vi "output.vi"(8 "error in":errorcluster, 10 "data table in":T1, 11 "FPGA Module runtime in":refnum<class "FPGA Module runtime.lvclass">) -> (0 "error out":errorcluster, 2 "data table out":T1, 3 "FPGA Module runtime out":refnum<class "FPGA Module runtime.lvclass">)   [LabVIEW 2017, in "FPGA Module runtime.lvclass"]
doc: "Provides an interface for writing data to a module at runtime. While this interface performs no operations, a child should provide an override which may write to any open sessions, references, or interfaces."
uses:
  FPGA Module runtime.lvclass
  <vilib>/NI/Tag Bus/table/data table.ctl
  FPGA Module runtime.lvclass/FPGA Module runtime.ctl
  OLD Project Folder/fpga channel/FXP I_20_5.ctl
  OLD Project Folder/fpga channel/FXP I_24_5.ctl
  OLD Project Folder/fpga channel/FXP I_24_10.ctl
  <vilib>/NI/Tag Bus/table/data polymorphs/read many/read Doubles.vi
  <vilib>/NI/Tag Bus/table/data polymorphs/read many/read Singles.vi
  <vilib>/NI/Tag Bus/table/data polymorphs/read many/read I64s.vi
  <vilib>/NI/Tag Bus/table/data polymorphs/read many/read I32s.vi
  <vilib>/NI/Tag Bus/table/data polymorphs/read many/read I16s.vi
  <vilib>/NI/Tag Bus/table/data polymorphs/read many/read I8s.vi
  <vilib>/NI/Tag Bus/table/data polymorphs/read many/read U64s.vi
  <vilib>/NI/Tag Bus/table/data polymorphs/read many/read U32s.vi
  <vilib>/NI/Tag Bus/table/data polymorphs/read many/read U16s.vi
  <vilib>/NI/Tag Bus/table/data polymorphs/read many/read U8s.vi
  <vilib>/NI/Tag Bus/table/data polymorphs/read many/read Booleans.vi
  <vilib>/NI/Tag Bus/table/data polymorphs/read many/read Array of Booleans.vi
  <vilib>/NI/Tag Bus/table/data polymorphs/read one/read Array of Double.vi
  <vilib>/NI/Tag Bus/table/data polymorphs/read one/read Array of Single.vi
  <vilib>/NI/Tag Bus/table/data polymorphs/read one/read Array of I64.vi
  <vilib>/NI/Tag Bus/table/data polymorphs/read one/read Array of I32.vi
  <vilib>/NI/Tag Bus/table/data polymorphs/read one/read Array of I16.vi
  <vilib>/NI/Tag Bus/table/data polymorphs/read one/read Array of I8.vi
  <vilib>/NI/Tag Bus/table/data polymorphs/read one/read Array of U64.vi
  <vilib>/NI/Tag Bus/table/data polymorphs/read one/read Array of U32.vi
  <vilib>/NI/Tag Bus/table/data polymorphs/read one/read Array of U16.vi
  <vilib>/NI/Tag Bus/table/data polymorphs/read one/read Array of U8.vi
  <vilib>/Utility/error.llb/Error Cluster From Error Code.vi
  <vilib>/rvi/errors/niLvFpgaAdjustHostInterfaceError.vi
  <vilib>/rvi/interface/nirviReadWriteControl/nirviReadWriteControl.xnode
  <vilib>/NI/Tag Bus/table/data table.lvlib
  fpga channel/FPGA Channel.lvclass
  NiFpgaLv.dll
  <vilib>/rvi/interface/Simulation/niFpgaSimulationCallBeginRW.vi
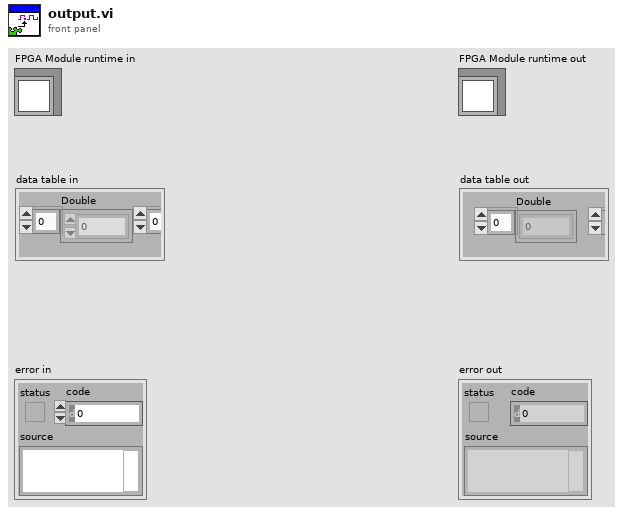
[diagram p1: front panel]
types:
  T1 = typedef "tag bus.lvlib/data table.lvlib/data table.ctl" = cluster{"Double":dbl[], "Single":sgl[], "I64":i64[], "I32":i32[], "I16":i16[], "I8":i8[], "U64":u64[], "U32":u32[], "U16":u16[], "U8":u8[], "Boolean":bool[], "String":string[], "Array of Double":cluster{"DBL Array":dbl[]}[], "Array of Single":cluster{"SGL Array":sgl[]}[], "Array of I64":cluster{"I64 Array":i64[]}[], "Array of I32":cluster{"I32 Array":i32[]}[], "Array of I16":cluster{"I16 Array":i16[]}[], "Array of I8":cluster{"I8 Array":i8[]}[], "Array of U64":cluster{"U64 Array":u64[]}[], "Array of U32":cluster{"U32 Array":u32[]}[], "Array of U16":cluster{"U16 Array":u16[]}[], "Array of U8":cluster{"U8 Array":u8[]}[], "Array of Boolean":cluster{"Boolean Array":bool[]}[], "Array of String":cluster{"String Array":string[]}[]}
  T2 = typedef "FPGA Module runtime.lvclass/ControlsMappings.ctl" = cluster{"data type":T3, "fpga res type":T4[], "fpga resource":refnum<k20>[], "data indexes":i32[]}
  T3 = typedef "tag bus.lvlib/tag descriptor.lvclass/Data Type.ctl" = enum16{"Double", "Single", "I64", "I32", "I16", "I8", "U64", "U32", "U16", "U8", "Boolean", "String", "Array of Double", "Array of Single", "Array of I64", "Array of I32", "Array of I16", "Array of I8", "Array of U64", "Array of U32", "Array of U16", "Array of U8", "Array of Boolean", "Array of String"}
  T4 = typedef "FPGA Channel.lvclass/fpga resource supported data types.ctl" = enum16{"Invalid Type", "Single", "I64", "I32", "I16", "I8", "U64", "U32", "U16", "U8", "Boolean", "FXP I,20,5", "FXP I,24,5", "FXP I,24,10", "Fifo 1023,I16"}
  T5 = typedef "FPGA Channel.lvclass/FXP I_20_5.ctl" = refnum<k20>
  T6 = typedef "FPGA Channel.lvclass/FXP I_24_5.ctl" = refnum<k20>
  T7 = typedef "FPGA Channel.lvclass/FXP I_24_10.ctl" = refnum<k20>
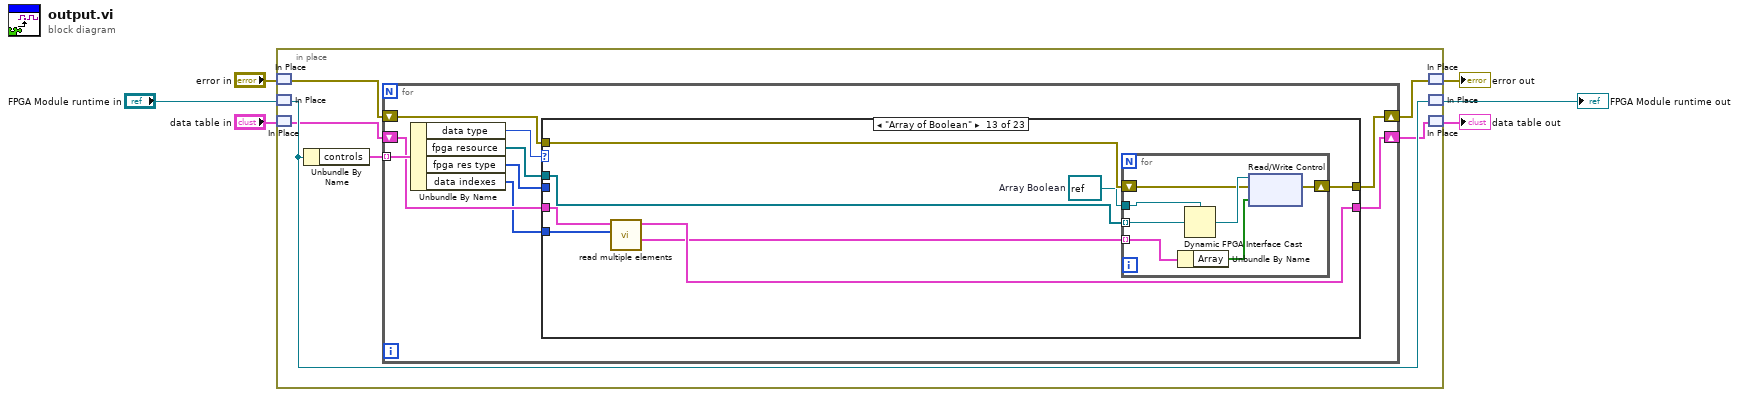
[diagram p0: block diagram]
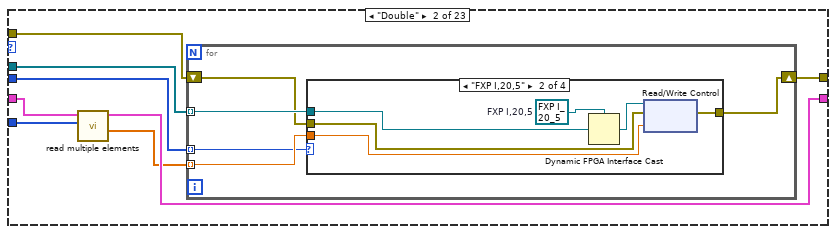
[diagram p3: hidden frame]
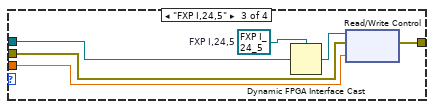
[diagram p5: hidden frame]
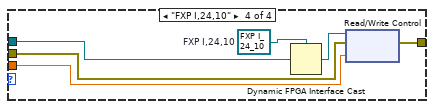
[diagram p6: hidden frame]
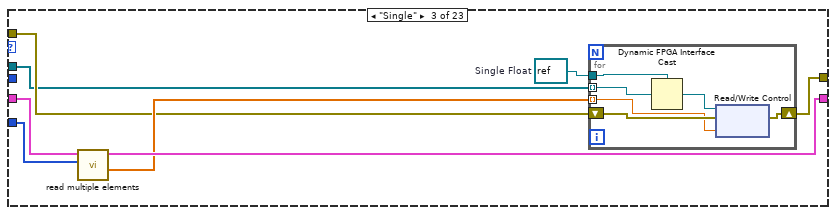
[diagram p7: hidden frame]
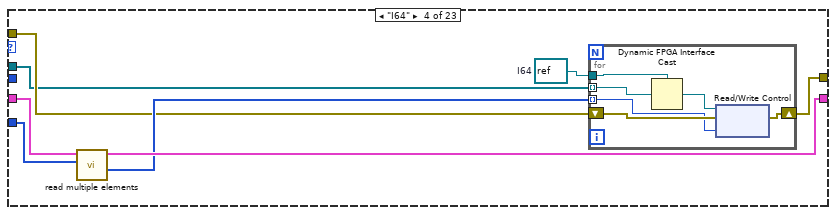
[diagram p8: hidden frame]
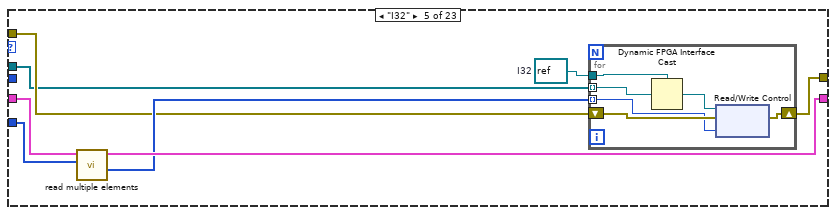
[diagram p9: hidden frame]
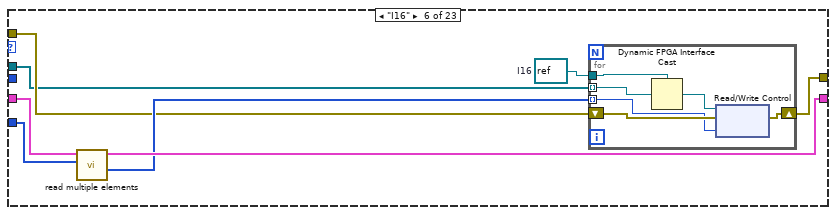
[diagram p10: hidden frame]
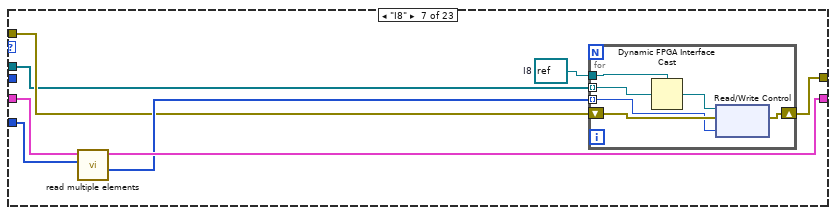
[diagram p11: hidden frame]
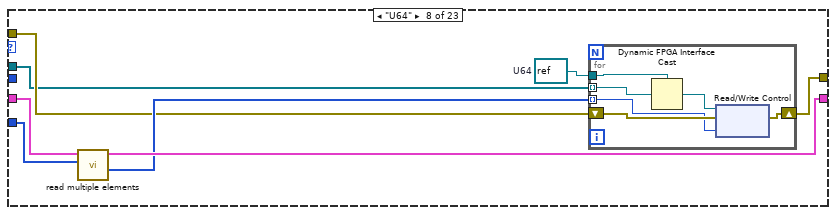
[diagram p12: hidden frame]
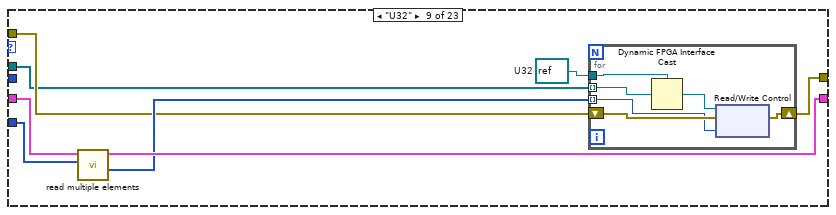
[diagram p13: hidden frame]
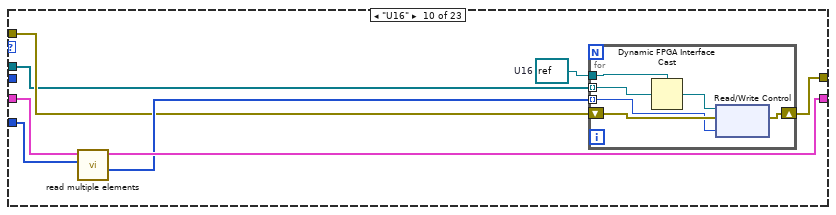
[diagram p14: hidden frame]
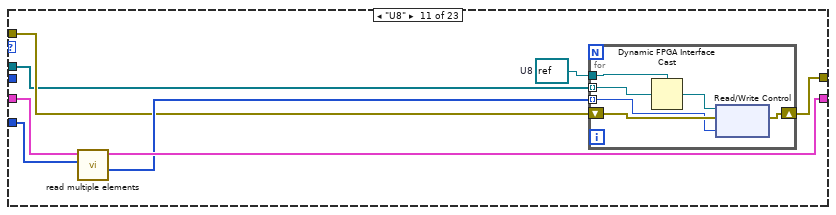
[diagram p15: hidden frame]
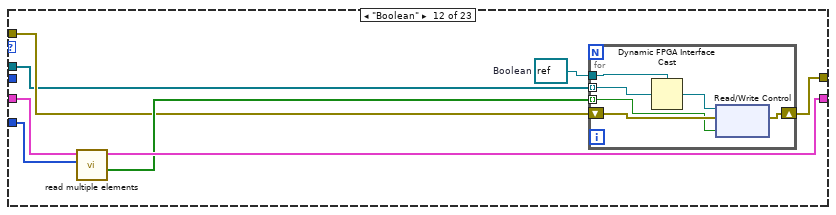
[diagram p16: hidden frame]
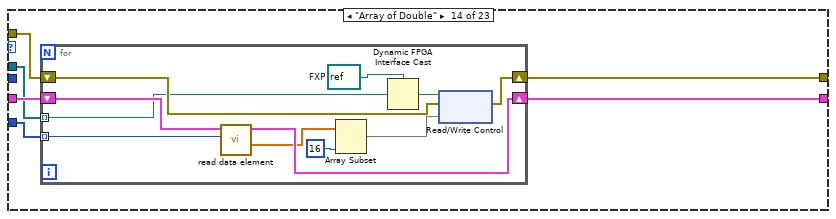
[diagram p17: hidden frame]
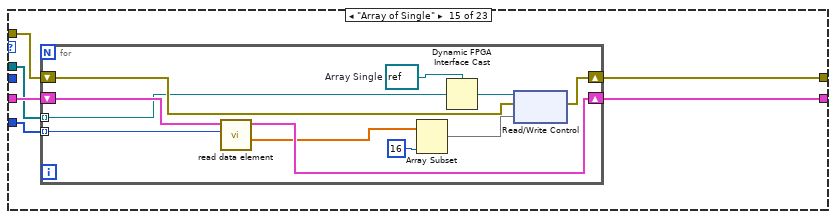
[diagram p18: hidden frame]
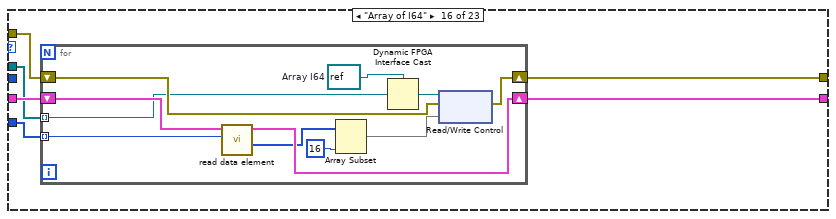
[diagram p19: hidden frame]
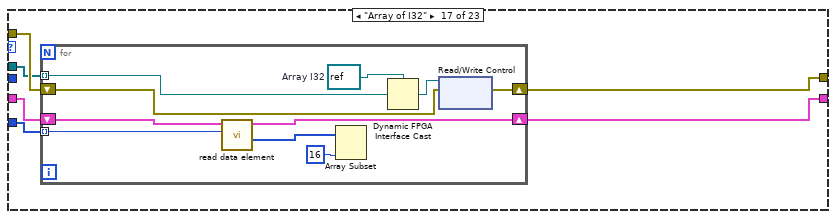
[diagram p20: hidden frame]
diagram:
  n1 = in-place {
    n2 = in-place-match #1("error in") -> (w7:errorcluster)
    n3 = in-place-match #2("FPGA Module runtime in") -> (w11:refnum<class "FPGA Module runtime.lvclass">)
    n4 = in-place-match #3("data table in") -> (w10:T1)
    n5 = Unbundle By Name(w11) -> ("controls"=w12:T2[])
    n6 = for {
      shift-right: [w20] -> w9
      shift-left: w10 -> [w19]
      shift-right: [w15] -> w8
      shift-left: w7 -> [w18]
      tunnel: w12 -> [w21] mode=indexing
      n7 = Unbundle By Name(w21) -> ("data type"=w14:T3, "fpga resource"=w16:refnum<k20>[], "fpga res type"=w13:T4[], "data indexes"=w17:i32[])
      n8 = case shown="\"Array of Boolean\"" w14 {
        tunnel: [w23 w30 w62 w76 w90 w104 w118 w132 w146 w160 w174 w188 w202 w215 w232 w249 w266 w282 w299 w316 w333 w350 w367] -> w20
        tunnel: w19 -> [w23 w31 w63 w77 w91 w105 w119 w133 w147 w161 w175 w189 w203 w216 w233 w250 w267 w283 w300 w317 w334 w351 w368]
        tunnel: w18 -> [w22 w27 w59 w73 w87 w101 w115 w129 w143 w157 w171 w185 w199 w213 w230 w247 w264 w280 w297 w314 w331 w348 w365]
        tunnel: w17 -> [_ w29 w61 w75 w89 w103 w117 w131 w145 w159 w173 w187 w201 w214 w231 w248 w265 w281 w298 w315 w332 w349 w366]
        tunnel: w16 -> [_ w26 w58 w72 w86 w100 w114 w128 w142 w156 w170 w184 w198 w212 w229 w246 w263 w279 w296 w313 w330 w347 w364]
        tunnel: [w22 w25 w56 w70 w84 w98 w112 w126 w140 w154 w168 w182 w197 w211 w228 w245 w262 w278 w295 w312 w329 w346 w363] -> w15
        tunnel: w13 -> [_ w24 _ _ _ _ _ _ _ _ _ _ _ _ _ _ _ _ _ _ _ _ _]
        frame Default {
        }
        frame "Double" {
          n9 = call-poly <vilib>:"read multiple elements.vi"("indices"=w29, "data table in"=w31) -> ("values"=w28:dbl[], "data table out"=w30:T1)  [unwired: 8 in]
          n10 = for {
            tunnel: w26 -> [w36] mode=indexing
            shift-right: [w34] -> w25
            shift-left: w27 -> [w35]
            tunnel: w28 -> [w33] mode=indexing
            tunnel: w24 -> [w32] mode=indexing
            n11 = case shown="\"FXP I,20,5\"" w32 {
              tunnel: w36 -> [_ w43 w49 w55]
              tunnel: w35 -> [w37 w41 w47 w53]
              tunnel: [w37 w40 w46 w52] -> w34
              tunnel: w33 -> [_ w39 w45 w51]
              frame "Invalid Type", Default {
              }
              frame "FXP I,20,5" {
                w38 = T5 refnum  # FXP I,20,5
                n12 = Dynamic FPGA Interface Cast(Session In=w38, Type=w43) -> (Session Out=w42:T5)
                n13 = xnode "Read/Write Control"("FPGA VI Reference In"=w42, "error in"=w41, "Value"=w39) -> ("error out"=w40:errorcluster)  [unwired: 1 out]
              }
              frame "FXP I,24,5" {
                w44 = T6 refnum  # FXP I,24,5
                n14 = Dynamic FPGA Interface Cast(Session In=w44, Type=w49) -> (Session Out=w48:T6)
                n15 = xnode "Read/Write Control"("FPGA VI Reference In"=w48, "error in"=w47, "Value"=w45) -> ("error out"=w46:errorcluster)  [unwired: 1 out]
              }
              frame "FXP I,24,10" {
                w50 = T7 refnum  # FXP I,24,10
                n16 = Dynamic FPGA Interface Cast(Session In=w50, Type=w55) -> (Session Out=w54:T7)
                n17 = xnode "Read/Write Control"("FPGA VI Reference In"=w54, "error in"=w53, "Value"=w51) -> ("error out"=w52:errorcluster)  [unwired: 1 out]
              }
            }
          }
        }
        frame "Single" {
          w57 = refnum<k20> refnum  # Single Float
          n18 = call-poly <vilib>:"read multiple elements.vi"("indices"=w61, "data table in"=w63) -> ("values"=w60:sgl[], "data table out"=w62:T1)  [unwired: 8 in]
          n19 = for {
            tunnel: w58 -> [w69] mode=indexing
            shift-right: [w66] -> w56
            shift-left: w59 -> [w67]
            tunnel: w57 -> [w65]
            tunnel: w60 -> [w64] mode=indexing
            n20 = Dynamic FPGA Interface Cast(Session In=w65, Type=w69) -> (Session Out=w68:refnum<k20>)
            n21 = xnode "Read/Write Control"("FPGA VI Reference In"=w68, "error in"=w67, "Value"=w64) -> ("error out"=w66:errorcluster)  [unwired: 1 out]
          }
        }
        frame "I64" {
          w71 = refnum<k20> refnum  # I64
          n22 = call-poly <vilib>:"read multiple elements.vi"("indices"=w75, "data table in"=w77) -> ("values"=w74:i64[], "data table out"=w76:T1)  [unwired: 8 in]
          n23 = for {
            tunnel: w72 -> [w83] mode=indexing
            shift-right: [w80] -> w70
            shift-left: w73 -> [w81]
            tunnel: w71 -> [w79]
            tunnel: w74 -> [w78] mode=indexing
            n24 = Dynamic FPGA Interface Cast(Session In=w79, Type=w83) -> (Session Out=w82:refnum<k20>)
            n25 = xnode "Read/Write Control"("FPGA VI Reference In"=w82, "error in"=w81, "Value"=w78) -> ("error out"=w80:errorcluster)  [unwired: 1 out]
          }
        }
        frame "I32" {
          w85 = refnum<k20> refnum  # I32
          n26 = call-poly <vilib>:"read multiple elements.vi"("indices"=w89, "data table in"=w91) -> ("values"=w88:i32[], "data table out"=w90:T1)  [unwired: 8 in]
          n27 = for {
            tunnel: w86 -> [w97] mode=indexing
            shift-right: [w94] -> w84
            shift-left: w87 -> [w95]
            tunnel: w85 -> [w93]
            tunnel: w88 -> [w92] mode=indexing
            n28 = Dynamic FPGA Interface Cast(Session In=w93, Type=w97) -> (Session Out=w96:refnum<k20>)
            n29 = xnode "Read/Write Control"("FPGA VI Reference In"=w96, "error in"=w95, "Value"=w92) -> ("error out"=w94:errorcluster)  [unwired: 1 out]
          }
        }
        frame "I16" {
          w99 = refnum<k20> refnum  # I16
          n30 = call-poly <vilib>:"read multiple elements.vi"("indices"=w103, "data table in"=w105) -> ("values"=w102:i16[], "data table out"=w104:T1)  [unwired: 8 in]
          n31 = for {
            tunnel: w100 -> [w111] mode=indexing
            shift-right: [w108] -> w98
            shift-left: w101 -> [w109]
            tunnel: w99 -> [w107]
            tunnel: w102 -> [w106] mode=indexing
            n32 = Dynamic FPGA Interface Cast(Session In=w107, Type=w111) -> (Session Out=w110:refnum<k20>)
            n33 = xnode "Read/Write Control"("FPGA VI Reference In"=w110, "error in"=w109, "Value"=w106) -> ("error out"=w108:errorcluster)  [unwired: 1 out]
          }
        }
        frame "I8" {
          w113 = refnum<k20> refnum  # I8
          n34 = call-poly <vilib>:"read multiple elements.vi"("indices"=w117, "data table in"=w119) -> ("values"=w116:i8[], "data table out"=w118:T1)  [unwired: 8 in]
          n35 = for {
            tunnel: w114 -> [w125] mode=indexing
            shift-right: [w122] -> w112
            shift-left: w115 -> [w123]
            tunnel: w113 -> [w121]
            tunnel: w116 -> [w120] mode=indexing
            n36 = Dynamic FPGA Interface Cast(Session In=w121, Type=w125) -> (Session Out=w124:refnum<k20>)
            n37 = xnode "Read/Write Control"("FPGA VI Reference In"=w124, "error in"=w123, "Value"=w120) -> ("error out"=w122:errorcluster)  [unwired: 1 out]
          }
        }
        frame "U64" {
          w127 = refnum<k20> refnum  # U64
          n38 = call-poly <vilib>:"read multiple elements.vi"("indices"=w131, "data table in"=w133) -> ("values"=w130:u64[], "data table out"=w132:T1)  [unwired: 8 in]
          n39 = for {
            tunnel: w128 -> [w139] mode=indexing
            shift-right: [w136] -> w126
            shift-left: w129 -> [w137]
            tunnel: w127 -> [w135]
            tunnel: w130 -> [w134] mode=indexing
            n40 = Dynamic FPGA Interface Cast(Session In=w135, Type=w139) -> (Session Out=w138:refnum<k20>)
            n41 = xnode "Read/Write Control"("FPGA VI Reference In"=w138, "error in"=w137, "Value"=w134) -> ("error out"=w136:errorcluster)  [unwired: 1 out]
          }
        }
        frame "U32" {
          w141 = refnum<k20> refnum  # U32
          n42 = call-poly <vilib>:"read multiple elements.vi"("indices"=w145, "data table in"=w147) -> ("values"=w144:u32[], "data table out"=w146:T1)  [unwired: 8 in]
          n43 = for {
            tunnel: w142 -> [w153] mode=indexing
            shift-right: [w150] -> w140
            shift-left: w143 -> [w151]
            tunnel: w141 -> [w149]
            tunnel: w144 -> [w148] mode=indexing
            n44 = Dynamic FPGA Interface Cast(Session In=w149, Type=w153) -> (Session Out=w152:refnum<k20>)
            n45 = xnode "Read/Write Control"("FPGA VI Reference In"=w152, "error in"=w151, "Value"=w148) -> ("error out"=w150:errorcluster)  [unwired: 1 out]
          }
        }
        frame "U16" {
          w155 = refnum<k20> refnum  # U16
          n46 = call-poly <vilib>:"read multiple elements.vi"("indices"=w159, "data table in"=w161) -> ("values"=w158:u16[], "data table out"=w160:T1)  [unwired: 8 in]
          n47 = for {
            tunnel: w156 -> [w167] mode=indexing
            shift-right: [w164] -> w154
            shift-left: w157 -> [w165]
            tunnel: w155 -> [w163]
            tunnel: w158 -> [w162] mode=indexing
            n48 = Dynamic FPGA Interface Cast(Session In=w163, Type=w167) -> (Session Out=w166:refnum<k20>)
            n49 = xnode "Read/Write Control"("FPGA VI Reference In"=w166, "error in"=w165, "Value"=w162) -> ("error out"=w164:errorcluster)  [unwired: 1 out]
          }
        }
        frame "U8" {
          w169 = refnum<k20> refnum  # U8
          n50 = call-poly <vilib>:"read multiple elements.vi"("indices"=w173, "data table in"=w175) -> ("values"=w172:u8[], "data table out"=w174:T1)  [unwired: 8 in]
          n51 = for {
            tunnel: w170 -> [w181] mode=indexing
            shift-right: [w178] -> w168
            shift-left: w171 -> [w179]
            tunnel: w169 -> [w177]
            tunnel: w172 -> [w176] mode=indexing
            n52 = Dynamic FPGA Interface Cast(Session In=w177, Type=w181) -> (Session Out=w180:refnum<k20>)
            n53 = xnode "Read/Write Control"("FPGA VI Reference In"=w180, "error in"=w179, "Value"=w176) -> ("error out"=w178:errorcluster)  [unwired: 1 out]
          }
        }
        frame "Boolean" {
          w183 = refnum<k20> refnum  # Boolean
          n54 = call-poly <vilib>:"read multiple elements.vi"("indices"=w187, "data table in"=w189) -> ("values"=w186:bool[], "data table out"=w188:T1)  [unwired: 8 in]
          n55 = for {
            tunnel: w184 -> [w195] mode=indexing
            shift-right: [w192] -> w182
            shift-left: w185 -> [w193]
            tunnel: w183 -> [w191]
            tunnel: w186 -> [w190] mode=indexing
            n56 = Dynamic FPGA Interface Cast(Session In=w191, Type=w195) -> (Session Out=w194:refnum<k20>)
            n57 = xnode "Read/Write Control"("FPGA VI Reference In"=w194, "error in"=w193, "Value"=w190) -> ("error out"=w192:errorcluster)  [unwired: 1 out]
          }
        }
        frame "Array of Boolean" {
          w196 = refnum<k20> refnum  # Array Boolean
          n58 = call-poly <vilib>:"read multiple elements.vi"("indices"=w201, "data table in"=w203) -> ("values"=w200:cluster{"Array":bool[]}[], "data table out"=w202:T1)  [unwired: 8 in]
          n59 = for {
            tunnel: w198 -> [w210] mode=indexing
            shift-right: [w207] -> w197
            shift-left: w199 -> [w208]
            tunnel: w196 -> [w206]
            tunnel: w200 -> [w205] mode=indexing
            n60 = Unbundle By Name(w205) -> ("Array"=w204:bool[])
            n61 = Dynamic FPGA Interface Cast(Session In=w206, Type=w210) -> (Session Out=w209:refnum<k20>)
            n62 = xnode "Read/Write Control"("FPGA VI Reference In"=w209, "error in"=w208, "Value"=w204) -> ("error out"=w207:errorcluster)  [unwired: 1 out]
          }
        }
        frame "Array of Double" {
          n63 = for {
            tunnel: w214 -> [w225] mode=indexing
            shift-right: [w226] -> w215
            shift-left: w216 -> [w227]
            tunnel: w212 -> [w221] mode=indexing
            shift-right: [w220] -> w211
            shift-left: w213 -> [w223]
            w222 = refnum<k20> refnum  # FXP
            n64 = call-poly <vilib>:"read data element.vi"("index"=w225, "data table in"=w227) -> ("value"=w219:dbl[], "data table out"=w226:T1)  [unwired: 8 in]
            n65 = Array Subset(array=w219, length=16) -> (w218:dbl[])  [unwired: 1 in]
            n66 = Dynamic FPGA Interface Cast(Session In=w222, Type=w221) -> (Session Out=w224:refnum<k20>)
            n67 = xnode "Read/Write Control"("FPGA VI Reference In"=w224, "error in"=w223, "Value"=w218) -> ("error out"=w220:errorcluster)  [unwired: 1 out]
          }
        }
        frame "Array of Single" {
          n68 = for {
            tunnel: w231 -> [w242] mode=indexing
            shift-right: [w243] -> w232
            shift-left: w233 -> [w244]
            tunnel: w229 -> [w239] mode=indexing
            shift-right: [w238] -> w228
            shift-left: w230 -> [w240]
            w236 = refnum<k20> refnum  # Array Single
            n69 = call-poly <vilib>:"read data element.vi"("index"=w242, "data table in"=w244) -> ("value"=w235:sgl[], "data table out"=w243:T1)  [unwired: 8 in]
            n70 = Array Subset(array=w235, length=16) -> (w234:sgl[])  [unwired: 1 in]
            n71 = Dynamic FPGA Interface Cast(Session In=w236, Type=w239) -> (Session Out=w241:refnum<k20>)
            n72 = xnode "Read/Write Control"("FPGA VI Reference In"=w241, "error in"=w240, "Value"=w234) -> ("error out"=w238:errorcluster)  [unwired: 1 out]
          }
        }
        frame "Array of I64" {
          n73 = for {
            tunnel: w248 -> [w259] mode=indexing
            shift-right: [w260] -> w249
            shift-left: w250 -> [w261]
            tunnel: w246 -> [w256] mode=indexing
            shift-right: [w255] -> w245
            shift-left: w247 -> [w257]
            w251 = refnum<k20> refnum  # Array I64
            n74 = call-poly <vilib>:"read data element.vi"("index"=w259, "data table in"=w261) -> ("value"=w254:i64[], "data table out"=w260:T1)  [unwired: 8 in]
            n75 = Array Subset(array=w254, length=16) -> (w253:i64[])  [unwired: 1 in]
            n76 = Dynamic FPGA Interface Cast(Session In=w251, Type=w256) -> (Session Out=w258:refnum<k20>)
            n77 = xnode "Read/Write Control"("FPGA VI Reference In"=w258, "error in"=w257, "Value"=w253) -> ("error out"=w255:errorcluster)  [unwired: 1 out]
          }
        }
        frame "Array of I32" {
          n78 = for {
            tunnel: w265 -> [w275] mode=indexing
            shift-right: [w276] -> w266
            shift-left: w267 -> [w277]
            tunnel: w263 -> [w272] mode=indexing
            shift-right: [w271] -> w262
            shift-left: w264 -> [w273]
            w268 = refnum<k20> refnum  # Array I32
            n79 = call-poly <vilib>:"read data element.vi"("index"=w275, "data table in"=w277) -> ("value"=w270:i32[], "data table out"=w276:T1)  [unwired: 8 in]
            n80 = Array Subset(array=w270, length=16) -> ()  [unwired: 1 in, 1 out]
            n81 = Dynamic FPGA Interface Cast(Session In=w268, Type=w272) -> (Session Out=w274:refnum<k20>)
            n82 = xnode "Read/Write Control"("FPGA VI Reference In"=w274, "error in"=w273) -> ("error out"=w271:errorcluster)  [unwired: 1 in, 1 out]
          }
        }
        frame "Array of I16" {
          n83 = for {
            tunnel: w281 -> [w292] mode=indexing
            shift-right: [w293] -> w282
            shift-left: w283 -> [w294]
            tunnel: w279 -> [w289] mode=indexing
            shift-right: [w288] -> w278
            shift-left: w280 -> [w290]
            w285 = refnum<k20> refnum  # Array I16
            n84 = call-poly <vilib>:"read data element.vi"("index"=w292, "data table in"=w294) -> ("value"=w287:i16[], "data table out"=w293:T1)  [unwired: 8 in]
            n85 = Array Subset(array=w287, length=16) -> (w284:i16[])  [unwired: 1 in]
            n86 = Dynamic FPGA Interface Cast(Session In=w285, Type=w289) -> (Session Out=w291:refnum<k20>)
            n87 = xnode "Read/Write Control"("FPGA VI Reference In"=w291, "error in"=w290, "Value"=w284) -> ("error out"=w288:errorcluster)  [unwired: 1 out]
          }
        }
        frame "Array of I8" {
          n88 = for {
            tunnel: w298 -> [w309] mode=indexing
            shift-right: [w310] -> w299
            shift-left: w300 -> [w311]
            tunnel: w296 -> [w306] mode=indexing
            shift-right: [w305] -> w295
            shift-left: w297 -> [w307]
            w301 = refnum<k20> refnum  # Array I8
            n89 = call-poly <vilib>:"read data element.vi"("index"=w309, "data table in"=w311) -> ("value"=w304:i8[], "data table out"=w310:T1)  [unwired: 8 in]
            n90 = Array Subset(array=w304, length=16) -> (w302:i8[])  [unwired: 1 in]
            n91 = Dynamic FPGA Interface Cast(Session In=w301, Type=w306) -> (Session Out=w308:refnum<k20>)
            n92 = xnode "Read/Write Control"("FPGA VI Reference In"=w308, "error in"=w307, "Value"=w302) -> ("error out"=w305:errorcluster)  [unwired: 1 out]
          }
        }
        frame "Array of U64" {
          n93 = for {
            tunnel: w315 -> [w326] mode=indexing
            shift-right: [w327] -> w316
            shift-left: w317 -> [w328]
            tunnel: w313 -> [w323] mode=indexing
            shift-right: [w322] -> w312
            shift-left: w314 -> [w324]
            w318 = refnum<k20> refnum  # Array U64
            n94 = call-poly <vilib>:"read data element.vi"("index"=w326, "data table in"=w328) -> ("value"=w321:u64[], "data table out"=w327:T1)  [unwired: 8 in]
            n95 = Array Subset(array=w321, length=16) -> (w319:u64[])  [unwired: 1 in]
            n96 = Dynamic FPGA Interface Cast(Session In=w318, Type=w323) -> (Session Out=w325:refnum<k20>)
            n97 = xnode "Read/Write Control"("FPGA VI Reference In"=w325, "error in"=w324, "Value"=w319) -> ("error out"=w322:errorcluster)  [unwired: 1 out]
          }
        }
        frame "Array of U32" {
          n98 = for {
            tunnel: w332 -> [w343] mode=indexing
            shift-right: [w344] -> w333
            shift-left: w334 -> [w345]
            tunnel: w330 -> [w340] mode=indexing
            shift-right: [w339] -> w329
            shift-left: w331 -> [w341]
            w335 = refnum<k20> refnum  # Array U32
            n99 = call-poly <vilib>:"read data element.vi"("index"=w343, "data table in"=w345) -> ("value"=w338:u32[], "data table out"=w344:T1)  [unwired: 8 in]
            n100 = Array Subset(array=w338, length=16) -> (w336:u32[])  [unwired: 1 in]
            n101 = Dynamic FPGA Interface Cast(Session In=w335, Type=w340) -> (Session Out=w342:refnum<k20>)
            n102 = xnode "Read/Write Control"("FPGA VI Reference In"=w342, "error in"=w341, "Value"=w336) -> ("error out"=w339:errorcluster)  [unwired: 1 out]
          }
        }
        frame "Array of U16" {
          n103 = for {
            tunnel: w349 -> [w360] mode=indexing
            shift-right: [w361] -> w350
            shift-left: w351 -> [w362]
            tunnel: w347 -> [w357] mode=indexing
            shift-right: [w356] -> w346
            shift-left: w348 -> [w358]
            w352 = refnum<k20> refnum  # Array U16
            n104 = call-poly <vilib>:"read data element.vi"("index"=w360, "data table in"=w362) -> ("value"=w355:u16[], "data table out"=w361:T1)  [unwired: 8 in]
            n105 = Array Subset(array=w355, length=16) -> (w353:u16[])  [unwired: 1 in]
            n106 = Dynamic FPGA Interface Cast(Session In=w352, Type=w357) -> (Session Out=w359:refnum<k20>)
            n107 = xnode "Read/Write Control"("FPGA VI Reference In"=w359, "error in"=w358, "Value"=w353) -> ("error out"=w356:errorcluster)  [unwired: 1 out]
          }
        }
        frame "Array of U8" {
          n108 = for {
            tunnel: w366 -> [w377] mode=indexing
            shift-right: [w378] -> w367
            shift-left: w368 -> [w379]
            tunnel: w364 -> [w374] mode=indexing
            shift-right: [w373] -> w363
            shift-left: w365 -> [w375]
            w369 = refnum<k20> refnum  # Array U8
            n109 = call-poly <vilib>:"read data element.vi"("index"=w377, "data table in"=w379) -> ("value"=w372:u8[], "data table out"=w378:T1)  [unwired: 8 in]
            n110 = Array Subset(array=w372, length=16) -> (w370:u8[])  [unwired: 1 in]
            n111 = Dynamic FPGA Interface Cast(Session In=w369, Type=w374) -> (Session Out=w376:refnum<k20>)
            n112 = xnode "Read/Write Control"("FPGA VI Reference In"=w376, "error in"=w375, "Value"=w370) -> ("error out"=w373:errorcluster)  [unwired: 1 out]
          }
        }
      }
    }
    n113 = in-place-match #1(w8) -> (→"error out":errorcluster)
    n114 = in-place-match #2(w11) -> (→"FPGA Module runtime out":refnum<class "FPGA Module runtime.lvclass">)
    n115 = in-place-match #3(w9) -> (→"data table out":T1)
  }
